vi "自动销毁句柄.vi"() -> ()   [LabVIEW 2011]
panel:
  out "引用句柄？":bool
  in  "x":bool
  in  "stop":bool
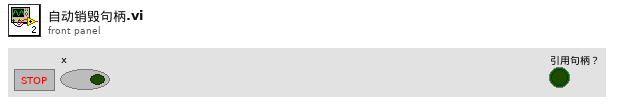
[diagram p1: front panel]
types:
  T1 = enum32{"Invalid", "Standard", "Closed", "Hidden", "Minimized", "Maximized"}
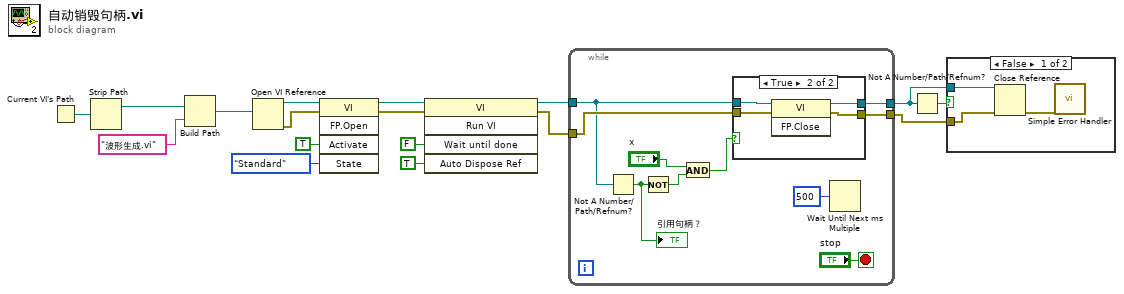
[diagram p0: block diagram]
diagram:
  n1 = Current VI's Path() -> (path=w17:path)
  n2 = Strip Path(path=w17) -> (stripped path=w16:path)  [unwired: 1 out]
  n3 = Build Path(base path=w16, name or relative path="波形生成.vi") -> (appended path=w14:path)
  n4 = Open VI Reference(vi path=w14) -> (vi reference=w13:refnum<vi>, error out=w12:errorcluster)  [unwired: 5 in]
  n5 = invoke class="VI" method="FP.Open"(reference=w13, error in=w12, "Activate"=TRUE ("Activate?"), "State"=T1."Standard") -> (reference out=w9:refnum<vi>, error out=w8:errorcluster)  [unwired: 1 in, 3 out]
  n6 = invoke class="VI" method="Run VI"(reference=w9, error in=w8, "Wait until done"=FALSE ("Wait Until Done"), "Auto Dispose Ref"=TRUE ("Auto Dispose Reference")) -> (reference out=w5:refnum<vi>, error out=w4:errorcluster)  [unwired: 1 in, 3 out]
  n7 = while {
    tunnel: w5 -> [w24]
    tunnel: w4 -> [w26]
    tunnel: [w25] -> w1
    tunnel: [w19] -> w2
    stop <- "stop" stop-if-true
    n8 = Not A Number/Path/Refnum?(number/path/refnum=w24) -> (NaN/Path/Refnum?=w23:bool)
    "引用句柄？" <- w23
    n9 = Not(x=w23) -> (.not. x?=w22:bool)
    n10 = And(x="x", y=w22) -> (x .and. y?=w21:bool)
    n11 = case shown="True" w21 {
      tunnel: w24 -> [w29 w33]
      tunnel: w26 -> [w28 w32]
      tunnel: [w29 w31] -> w19
      tunnel: [w28 w30] -> w25
      frame False {
      }
      frame True {
        n12 = invoke class="VI" method="FP.Close"(reference=w33, error in=w32) -> (reference out=w31:refnum<vi>, error out=w30:errorcluster)  [unwired: 1 in, 1 out]
      }
    }
    n13 = Wait Until Next ms Multiple(millisecond multiple=u32 500) -> ()  [unwired: 1 out]
  }
  n14 = Not A Number/Path/Refnum?(number/path/refnum=w2) -> (NaN/Path/Refnum?=w3:bool)
  n15 = case shown="False" w3 {
    tunnel: w2 -> [w36 _]
    tunnel: w1 -> [w35 _]
    frame False {
      n16 = Close Reference(reference=w36, error in (no error)=w35) -> (error out=w34:errorcluster)
      n17 = call <vilib>:"Simple Error Handler.vi"("error in (no error)"=w34) -> ()  [unwired: 4 in, 5 out]
    }
    frame True {
    }
  }
